vi "word2float.vi"(1 "Tableau d'entrée":u16[](array[numeric])) -> (0 "Float de sortie":sgl)   [LabVIEW 2019]
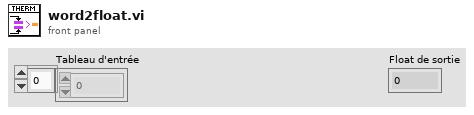
[diagram p1: front panel]
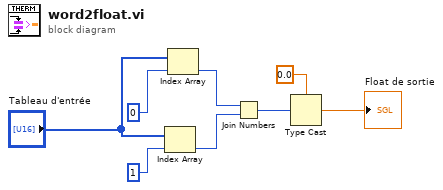
[diagram p0: block diagram]
diagram:
  n1 = Index Array(array="Tableau d'entrée", index=1 ("indice")) -> (element=w3:u16)
  n2 = Index Array(array="Tableau d'entrée", index=0 ("indice")) -> (element=w8:u16)
  n3 = Join Numbers(hi=w8, lo=w3) -> ((hi.lo)=w1:u32)
  n4 = Type Cast(type=sgl 0.0 ("starting address"), x=w1) -> (*(type *) &x=→"Float de sortie":sgl)
